vi "Temperature viewer.vi"(3 "ChipID+T array":u32[](array[numeric]) format="%.0x") -> ()   [LabVIEW 2015, in "VIPM2.lvlib"]
uses:
  VIPM2.lvlib
panel:
  out "S18 Chart":sgl(graph)
  out "S18 histogram":T1(graph) caption="Temperature histogram"
  out "S17 Chart":sgl(graph)
  out "S17 histogram":T1(graph) caption="Temperature histogram"
  out "S16 Chart":sgl(graph)
  out "S16 histogram":T1(graph) caption="Temperature histogram"
  out "S15 Chart":sgl(graph)
  out "S15 histogram":T1(graph) caption="Temperature histogram"
  out "S14 Chart":sgl(graph)
  out "S14 histogram":T1(graph) caption="Temperature histogram"
  out "S13 Chart":sgl(graph)
  out "S13 histogram":T1(graph) caption="Temperature histogram"
  out "S12 Chart":sgl(graph)
  out "S12 histogram":T1(graph) caption="Temperature histogram"
  out "S11 Chart":sgl(graph)
  out "S11 histogram":T1(graph) caption="Temperature histogram"
  out "S10 Chart":sgl(graph)
  out "S10 histogram":T1(graph) caption="Temperature histogram"
  out "S09 Chart":sgl(graph)
  out "S09 histogram":T1(graph) caption="Temperature histogram"
  out "S08 Chart":sgl(graph)
  out "S08 histogram":T1(graph) caption="Temperature histogram"
  out "S07 Chart":sgl(graph)
  out "S07 histogram":T1(graph) caption="Temperature histogram"
  out "S06 Chart":sgl(graph)
  out "S06 histogram":T1(graph) caption="Temperature histogram"
  out "S05 Chart":sgl(graph)
  out "S05 histogram":T1(graph) caption="Temperature histogram"
  out "S04 Chart":sgl(graph)
  out "S04 histogram":T1(graph) caption="Temperature histogram"
  out "S03 Chart":sgl(graph)
  out "S03 histogram":T1(graph) caption="Temperature histogram"
  out "S02 Chart":sgl(graph)
  out "S02 histogram":T1(graph) caption="Temperature histogram"
  out "S01 Chart":sgl(graph)
  out "S01 histogram":T1(graph) caption="Temperature histogram"
  # "Sector 01"
  # "Sector 02"
  # "Sector 03"
  # "Sector 04"
  # "Sector 05"
  # "Sector 06"
  # "Sector 07"
  # "Sector 08"
  # "Sector 09"
  # "Sector 10"
  # "Sector 11"
  # "Sector 12"
  # "Sector 13"
  # "Sector 14"
  # "Sector 15"
  # "Sector 16"
  # "Sector 17"
  # "Sector 18"
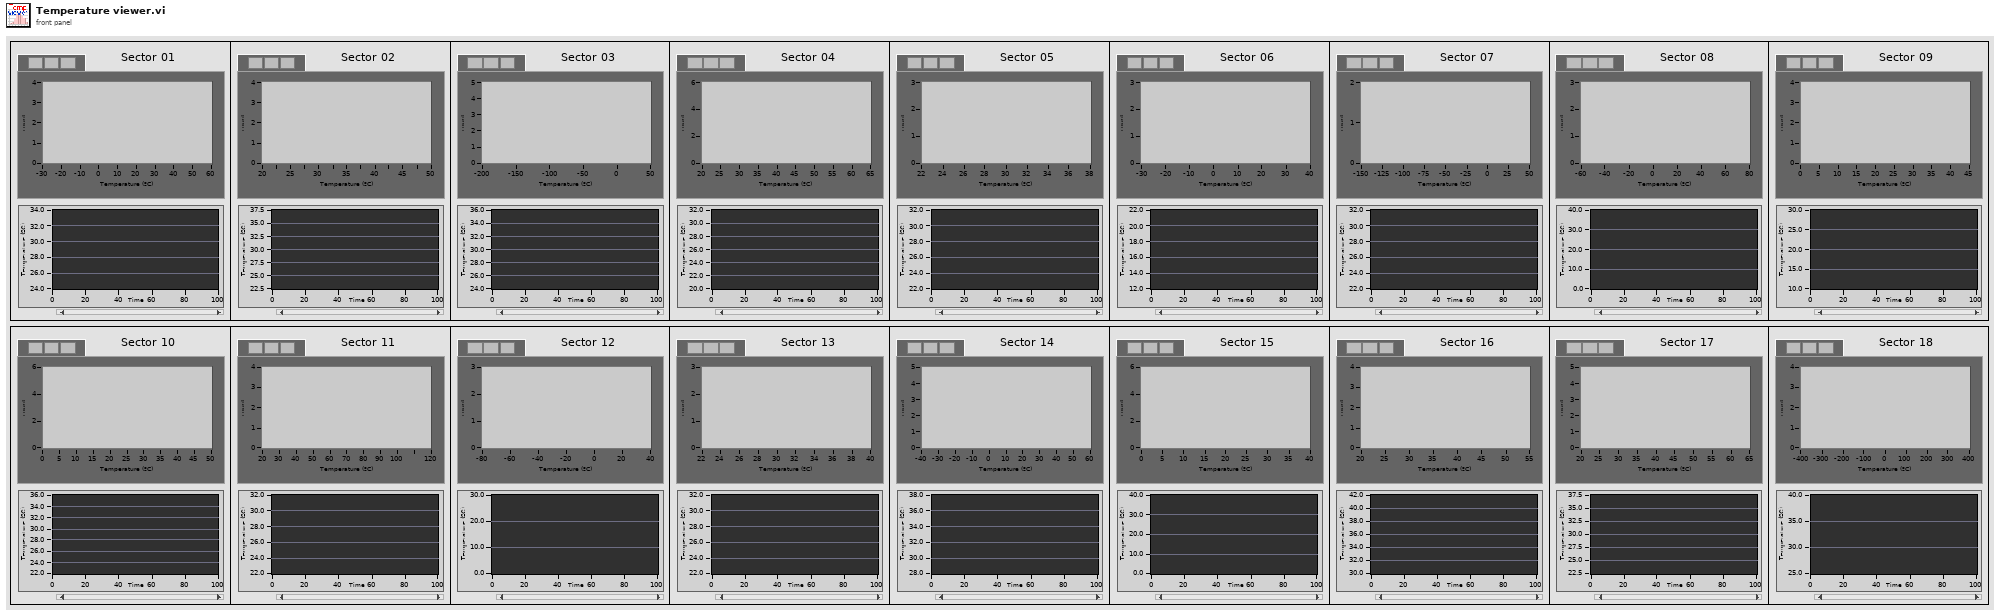
[diagram p1: front panel]
types:
  T1 = cluster{"X Values":dbl[], "Histogram: h(x)":i32[]}
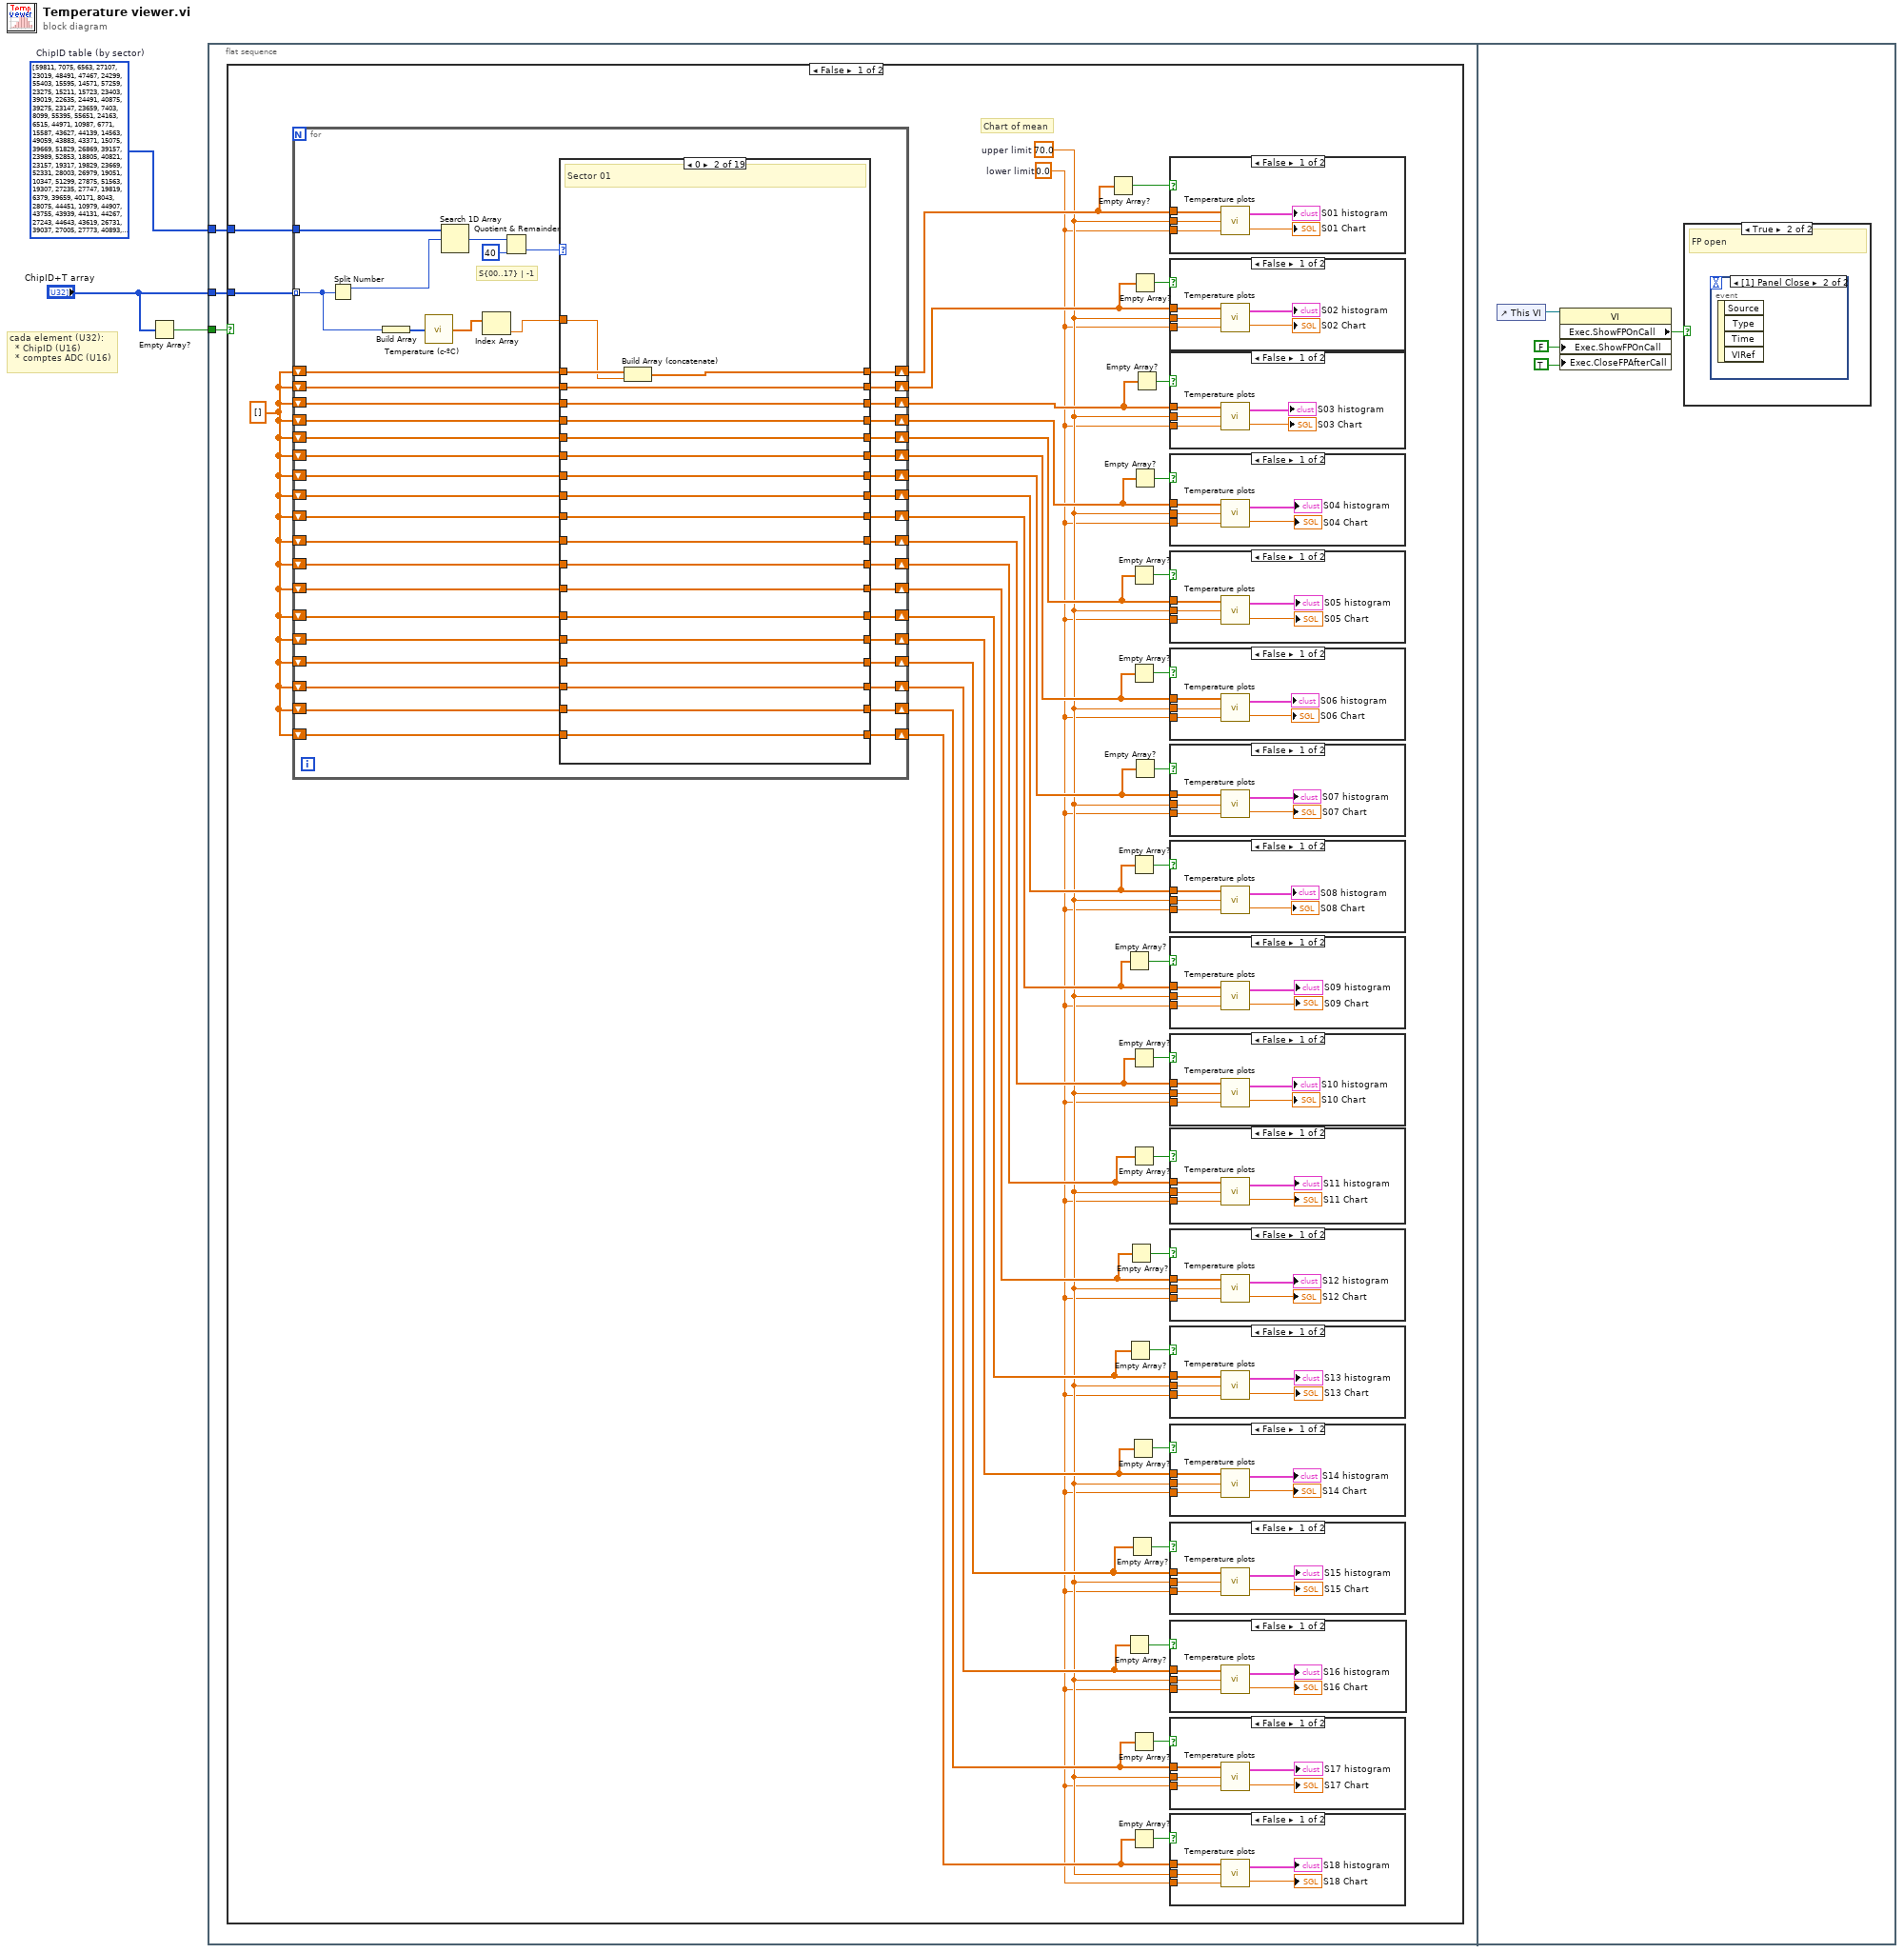
[diagram p0: block diagram]
diagram:
  w2 = u16[] [59811, 7075, 6563, 27107, 23019, 48491, 47467, 24299, 55403, 15595, 14571, 57259, 23275, 15211, 15723, 23403, 39019, 22635, 24491, 40875, 39275, 23147, 23659, 7403, 8099, 55395, 55651, 24163, 6515, 44971, 10987, 6771, 15587, 43627, 44139, 14563, 49059, 43883, 43371, 15075, 39669, 51829, 26869, 39157, 23989, 52853, 18805, 40821, 23157, 19317, 19829, 23669, 52331, 28003, 26979, 19051, 10347, 51299, 27875, 51563, 19307, 27235, 27747, 19819, 6379, 39659, 40171, 8043, 28075, 44451, 10979, 44907, 43755, 43939, 44131, 44267, 27243, 44643, 43619, 26731, 39037, 27005, 27773, 40893, 40189, 27517, 28029, 39165, 56165, 60645, 59621, 56677, 55525, 60261, 60517, 57189, 48357, 60773, 61349, 47333, 61309, 14461, 16317, 60797, 6525, 14965, 24189, 8125, 31845, 7781, 8101, 47845, 60669, 55805, 56061, 59773, 47973, 6245, 61157, 16229, 60541, 56765, 23037, 59517, 6589, 56445, 57277, 59901, 61181, 55549, 57213, 61373, 23485, 28285, 43133, 23997, 23677, 43965, 44477, 24509, 26877, 23293, 23805, 28541, 6765, 57261, 23789, 7085, 6509, 56941, 55917, 7789, 43629, 56045, 55661, 7533, 39421, 27581, 44925, 40317, 44269, 15469, 16301, 43245, 22627, 43261, 43645, 23971, 39549, 43389, 44669, 8035, 39293, 43773, 44285, 40573, 27885, 15603, 14579, 26861, 19309, 49075, 15731, 19821, 52845, 31859, 47859, 18797, 16125, 40867, 39843, 15101, 40675, 7421, 6397, 40291, 40163, 7037, 44157, 40803, 60269, 23021, 23405, 60781, 60141, 22765, 56429, 61293, 40805, 15741, 14717, 40037, 40165, 47869, 48381, 39141, 40677, 30973, 16253, 39653, 23141, 40035, 32381, 23461, 8037, 40547, 39523, 7013, 15613, 7907, 6883, 15997, 44397, 56173, 56685, 43373, 44909, 15277, 55789, 11501, 51835, 20071, 11003, 20091, 11195, 10491, 11131, 52603, 51451, 11643, 10619, 53115, 40827, 27239, 28263, 47207, 39291, 43111, 28071, 39803, 40059, 44391, 43879, 39547, 44661, 52469, 19061, 43637, 43957, 51445, 53109, 44469, 10997, 52597, 51573, 39797, 31341, 61037, 60013, 31853, 61051, 6267, 8123, 60027, 39867, 43623, 44647, 39035, 40379, 11495, 44135, 7931, 8059, 44455, 43943, 6395, 59835, 7099, 6587, 61371, 27131, 60155, 59899, 27387, 6375, 39655, 48359, 8039, 47847, 31335, 32359, 47335, 15975, 48743, 1120, 14951, 15719, 15079, 14567, 14695, 43387, 28282, 27259, 44667, 43899, 28027, 27003, 44411, 52333, 14949, 47347, 51309, 15973, 11879, 11367, 96, 31589, 60325, 60837, 31333, 14565, 15589, 15205, 14693, 43259, 28539, 27515, 44923, 3879, 57191, 56167, 57255, 55527, 56551, 15271, 14439, 31591, 23271, 23783, 31079, 60795, 7803, 6779, 59771, 61307, 7547, 6523, 60283, 26983, 61287, 59879, 28007, 26727, 6567, 8103, 26855, 59623, 7271, 39163, 59815, 40359, 23975, 39399, 39335, 40551, 22631, 24487, 39783, 39847, 23655, 23143, 39271, 60519, 40187, 39675, 60007, 27367, 24507, 23675, 60263, 27499, 44387, 43363, 26987, 26859, 28579, 44899, 28523, 57203, 39155, 40819, 56179, 56563, 39667, 40179, 55539, 15283, 39411, 40691, 57075, 56939, 47339, 48235, 56747, 55531, 31851, 48363, 56171, 44987, 43771, 44283, 43963, 43643, 28091, 26747, 44155, 15275, 31083, 32363, 55787, 59827, 48355, 47331, 27123, 61043, 31843, 47843, 60019, 60323, 7267, 6243, 60835, 59491, 6499, 7779, 27363, 39787, 59755, 61035, 40299, 23267, 56675, 57187, 23395, 22755, 55523, 56035, 24419, 55715, 57059, 40811, 24291, 23781, 56037, 56549, 22885, 39845, 48765, 47741, 416, 60147, 31075, 48995, 60659, 15725, 10365, 12221, 14701, 47213, 11197, 51453, 49069, 19815, 10343, 52455, 18791, 52071, 11111, 11623, 52839, 39269, 47997, 48509, 40549, 7525, 49021, 48253, 6501, 40373, 26741, 28597, 39349, 40885, 43893, 43381, 39861, 39285, 28021, 44917, 40053, 15597, 11133, 10877, 14957, 51437, 49011, 48243, 53101, 10605, 48755, 47731, 11885, 31603, 57267, 23795, 32115, 56755, 39795, 40307, 24307, 55667, 23475, 60339, 55923, 11637, 32109, 31085, 10613, 12149, 52093, 31597, 11125, 16237, 19325, 18813, 15213, 6387, 22643, 24499, 14451, 7923, 23155, 23667, 6899, 16227, 47459, 48739, 14691, 10477, 47987, 47219, 12141, 24435, 40369, 39347, 23411, 31091, 30963, 32627, 32371, 47981, 10621, 11901, 48493, 47341, 10493, 12157, 48237, 47853, 60845, 27373, 48365, 31349, 15285, 55797, 31861, 60661, 56949, 55925, 59637, 59765, 56053, 55669, 48373, 60341, 56693, 23797, 60853, 59509, 23029, 24309, 61365, 60277, 23925, 23413, 60789, 31093, 6261, 60533, 32373, 31605, 6517, 6773, 32117, 30965, 15477, 14453, 32629, 7925, 44277, 43253, 6901, 40363, 39403, 40683, 39339, 6581, 7029, 8053, 59893, 60349, 47349, 49013, 6269, 27133, 16117, 48757, 27389, 24445, 47989, 47221, 23933, 26867, 31587, 32099, 60787, 7091, 30947, 32611, 59891, 7539, 47203, 11499, 6259, 28013, 16243, 15219, 26989, 28525, 14963, 11117, 28589, 28077, 12205, 52461, 27245, 55909, 61029, 60005, 57253, 23397, 14437, 16293, 23909, 55653, 60133, 59749, 56933, 10475, 51811, 19043, 11883, 10859, 52067, 51555, 11491, 51427, 60003, 60515, 52451, 23915, 14699, 15979, 22891, 60331, 16107, 15459, 61291, 39531, 60139, 60651, 40043, 10595, 60643, 59619, 11875, 11363, 60259, 61027, 12195]  # ChipID table (by sector)
  # "cada element (U32):\n  * ChipID (U16)\n  * comptes ADC (U16)"
  n1 = Empty Array?(array="ChipID+T array") -> (empty?=w1:bool)
  n2 = flat-sequence {
    tunnel: "ChipID+T array" -> [w6]
    tunnel: w2 -> [w5]
    tunnel: w1 -> [w4]
    frame #0 {
      n3 = case shown="False" w4 {
        tunnel: w6 -> [w47 _]
        tunnel: w5 -> [w46 _]
        frame False {
          w8 = sgl 70.0  # upper limit
          w7 = sgl 0.0  # lower limit
          w42 = sgl[] []
          # "Chart of mean"
          n4 = for {
            tunnel: w47 -> [w141] mode=indexing
            tunnel: w46 -> [w181]
            shift-right: [w179] -> w45
            shift-left: w42 -> [w180]
            shift-right: [w174] -> w41
            shift-left: w42 -> [w178]
            shift-right: [w173] -> w39
            shift-left: w42 -> [w177]
            shift-right: [w172] -> w37
            shift-left: w42 -> [w176]
            shift-right: [w171] -> w35
            shift-left: w42 -> [w175]
            shift-right: [w154] -> w33
            shift-left: w42 -> [w167]
            shift-right: [w153] -> w31
            shift-left: w42 -> [w166]
            shift-right: [w152] -> w29
            shift-left: w42 -> [w165]
            shift-right: [w151] -> w27
            shift-left: w42 -> [w164]
            shift-right: [w150] -> w25
            shift-left: w42 -> [w163]
            shift-right: [w149] -> w23
            shift-left: w42 -> [w162]
            shift-right: [w148] -> w21
            shift-left: w42 -> [w161]
            shift-right: [w147] -> w19
            shift-left: w42 -> [w160]
            shift-right: [w146] -> w17
            shift-left: w42 -> [w159]
            shift-right: [w145] -> w15
            shift-left: w42 -> [w158]
            shift-right: [w144] -> w13
            shift-left: w42 -> [w157]
            shift-right: [w143] -> w11
            shift-left: w42 -> [w156]
            shift-right: [w142] -> w9
            shift-left: w42 -> [w155]
            # "S{00..17} | -1"
            n5 = Split Number(x=w141) -> (hi(x)=w182:u16)  [unwired: 1 out]
            n6 = Build Array(w141) -> (w140:u32[])
            n7 = call "Temperature (c-ºC).vi"("ChipID + Tcounts"=w140) -> ("Temperatures in ºC"=w139:sgl[])  [unwired: 3 in]
            n8 = Search 1D Array(1D array=w181, element=w182) -> (index of element=w170:i32)  [unwired: 1 in]
            n9 = Index Array(array=w139) -> (element=w138:sgl)  [unwired: 1 in]
            n10 = Quotient & Remainder(x=w170, y=40) -> (floor(x/y)=w168:i32)  [unwired: 1 out]
            n11 = case shown="0" w168 {
              tunnel: w138 -> [_ w219 w238 w257 w276 w295 w314 w333 w352 w371 w390 w409 w428 w447 w466 w485 w504 w523 w542]
              tunnel: w180 -> [w200 w220 w240 w260 w280 w300 w320 w340 w360 w380 w400 w420 w440 w460 w480 w500 w520 w540 w560]
              tunnel: [w200 w218 w240 w260 w280 w300 w320 w340 w360 w380 w400 w420 w440 w460 w480 w500 w520 w540 w560] -> w179
              tunnel: w178 -> [w199 w217 w239 w259 w279 w299 w319 w339 w359 w379 w399 w419 w439 w459 w479 w499 w519 w539 w559]
              tunnel: w177 -> [w198 w216 w236 w258 w278 w298 w318 w338 w358 w378 w398 w418 w438 w458 w478 w498 w518 w538 w558]
              tunnel: w176 -> [w197 w215 w235 w255 w277 w297 w317 w337 w357 w377 w397 w417 w437 w457 w477 w497 w517 w537 w557]
              tunnel: w175 -> [w196 w214 w234 w254 w274 w296 w316 w336 w356 w376 w396 w416 w436 w456 w476 w496 w516 w536 w556]
              tunnel: [w199 w217 w237 w259 w279 w299 w319 w339 w359 w379 w399 w419 w439 w459 w479 w499 w519 w539 w559] -> w174
              tunnel: [w198 w216 w236 w256 w278 w298 w318 w338 w358 w378 w398 w418 w438 w458 w478 w498 w518 w538 w558] -> w173
              tunnel: [w197 w215 w235 w255 w275 w297 w317 w337 w357 w377 w397 w417 w437 w457 w477 w497 w517 w537 w557] -> w172
              tunnel: [w196 w214 w234 w254 w274 w294 w316 w336 w356 w376 w396 w416 w436 w456 w476 w496 w516 w536 w556] -> w171
              tunnel: w167 -> [w195 w213 w233 w253 w273 w293 w315 w335 w355 w375 w395 w415 w435 w455 w475 w495 w515 w535 w555]
              tunnel: w166 -> [w194 w212 w232 w252 w272 w292 w312 w334 w354 w374 w394 w414 w434 w454 w474 w494 w514 w534 w554]
              tunnel: w165 -> [w193 w211 w231 w251 w271 w291 w311 w331 w353 w373 w393 w413 w433 w453 w473 w493 w513 w533 w553]
              tunnel: w164 -> [w192 w210 w230 w250 w270 w290 w310 w330 w350 w372 w392 w412 w432 w452 w472 w492 w512 w532 w552]
              tunnel: w163 -> [w191 w209 w229 w249 w269 w289 w309 w329 w349 w369 w391 w411 w431 w451 w471 w491 w511 w531 w551]
              tunnel: w162 -> [w190 w208 w228 w248 w268 w288 w308 w328 w348 w368 w388 w410 w430 w450 w470 w490 w510 w530 w550]
              tunnel: w161 -> [w189 w207 w227 w247 w267 w287 w307 w327 w347 w367 w387 w407 w429 w449 w469 w489 w509 w529 w549]
              tunnel: w160 -> [w188 w206 w226 w246 w266 w286 w306 w326 w346 w366 w386 w406 w426 w448 w468 w488 w508 w528 w548]
              tunnel: w159 -> [w187 w205 w225 w245 w265 w285 w305 w325 w345 w365 w385 w405 w425 w445 w467 w487 w507 w527 w547]
              tunnel: w158 -> [w186 w204 w224 w244 w264 w284 w304 w324 w344 w364 w384 w404 w424 w444 w464 w486 w506 w526 w546]
              tunnel: w157 -> [w185 w203 w223 w243 w263 w283 w303 w323 w343 w363 w383 w403 w423 w443 w463 w483 w505 w525 w545]
              tunnel: w156 -> [w184 w202 w222 w242 w262 w282 w302 w322 w342 w362 w382 w402 w422 w442 w462 w482 w502 w524 w544]
              tunnel: w155 -> [w183 w201 w221 w241 w261 w281 w301 w321 w341 w361 w381 w401 w421 w441 w461 w481 w501 w521 w543]
              tunnel: [w195 w213 w233 w253 w273 w293 w313 w335 w355 w375 w395 w415 w435 w455 w475 w495 w515 w535 w555] -> w154
              tunnel: [w194 w212 w232 w252 w272 w292 w312 w332 w354 w374 w394 w414 w434 w454 w474 w494 w514 w534 w554] -> w153
              tunnel: [w193 w211 w231 w251 w271 w291 w311 w331 w351 w373 w393 w413 w433 w453 w473 w493 w513 w533 w553] -> w152
              tunnel: [w192 w210 w230 w250 w270 w290 w310 w330 w350 w370 w392 w412 w432 w452 w472 w492 w512 w532 w552] -> w151
              tunnel: [w191 w209 w229 w249 w269 w289 w309 w329 w349 w369 w389 w411 w431 w451 w471 w491 w511 w531 w551] -> w150
              tunnel: [w190 w208 w228 w248 w268 w288 w308 w328 w348 w368 w388 w408 w430 w450 w470 w490 w510 w530 w550] -> w149
              tunnel: [w189 w207 w227 w247 w267 w287 w307 w327 w347 w367 w387 w407 w427 w449 w469 w489 w509 w529 w549] -> w148
              tunnel: [w188 w206 w226 w246 w266 w286 w306 w326 w346 w366 w386 w406 w426 w446 w468 w488 w508 w528 w548] -> w147
              tunnel: [w187 w205 w225 w245 w265 w285 w305 w325 w345 w365 w385 w405 w425 w445 w465 w487 w507 w527 w547] -> w146
              tunnel: [w186 w204 w224 w244 w264 w284 w304 w324 w344 w364 w384 w404 w424 w444 w464 w484 w506 w526 w546] -> w145
              tunnel: [w185 w203 w223 w243 w263 w283 w303 w323 w343 w363 w383 w403 w423 w443 w463 w483 w503 w525 w545] -> w144
              tunnel: [w184 w202 w222 w242 w262 w282 w302 w322 w342 w362 w382 w402 w422 w442 w462 w482 w502 w522 w544] -> w143
              tunnel: [w183 w201 w221 w241 w261 w281 w301 w321 w341 w361 w381 w401 w421 w441 w461 w481 w501 w521 w541] -> w142
              frame -1, Default {
                # "ChipID not found"
              }
              frame 0 {
                # "Sector 01"
                n12 = Build Array (concatenate) "Build Array"(w220, w219) -> (w218:sgl[])
              }
              frame 1 {
                # "Sector 02"
                n13 = Build Array (concatenate)(w239, w238) -> (w237:sgl[])
              }
              frame 2 {
                # "Sector 03"
                n14 = Build Array (concatenate)(w258, w257) -> (w256:sgl[])
              }
              frame 3 {
                # "Sector 04"
                n15 = Build Array (concatenate)(w277, w276) -> (w275:sgl[])
              }
              frame 4 {
                # "Sector 05"
                n16 = Build Array (concatenate)(w296, w295) -> (w294:sgl[])
              }
              frame 5 {
                # "Sector 06"
                n17 = Build Array (concatenate)(w315, w314) -> (w313:sgl[])
              }
              frame 6 {
                # "Sector 07"
                n18 = Build Array (concatenate)(w334, w333) -> (w332:sgl[])
              }
              frame 7 {
                # "Sector 08"
                n19 = Build Array (concatenate)(w353, w352) -> (w351:sgl[])
              }
              frame 8 {
                # "Sector 09"
                n20 = Build Array (concatenate)(w372, w371) -> (w370:sgl[])
              }
              frame 9 {
                # "Sector 10"
                n21 = Build Array (concatenate)(w391, w390) -> (w389:sgl[])
              }
              frame 10 {
                # "Sector 11"
                n22 = Build Array (concatenate)(w410, w409) -> (w408:sgl[])
              }
              frame 11 {
                # "Sector 12"
                n23 = Build Array (concatenate)(w429, w428) -> (w427:sgl[])
              }
              frame 12 {
                # "Sector 13"
                n24 = Build Array (concatenate)(w448, w447) -> (w446:sgl[])
              }
              frame 13 {
                # "Sector 14"
                n25 = Build Array (concatenate)(w467, w466) -> (w465:sgl[])
              }
              frame 14 {
                # "Sector 15"
                n26 = Build Array (concatenate)(w486, w485) -> (w484:sgl[])
              }
              frame 15 {
                # "Sector 16"
                n27 = Build Array (concatenate)(w505, w504) -> (w503:sgl[])
              }
              frame 16 {
                # "Sector 17"
                n28 = Build Array (concatenate)(w524, w523) -> (w522:sgl[])
              }
              frame 17 {
                # "Sector 18"
                n29 = Build Array (concatenate)(w543, w542) -> (w541:sgl[])
              }
            }
          }
          n30 = Empty Array?(array=w45) -> (empty?=w44:bool)
          n31 = Empty Array?(array=w27) -> (empty?=w28:bool)
          n32 = Empty Array?(array=w13) -> (empty?=w14:bool)
          n33 = Empty Array?(array=w19) -> (empty?=w20:bool)
          n34 = Empty Array?(array=w21) -> (empty?=w22:bool)
          n35 = Empty Array?(array=w15) -> (empty?=w16:bool)
          n36 = Empty Array?(array=w17) -> (empty?=w18:bool)
          n37 = Empty Array?(array=w35) -> (empty?=w36:bool)
          n38 = Empty Array?(array=w33) -> (empty?=w34:bool)
          n39 = Empty Array?(array=w29) -> (empty?=w30:bool)
          n40 = Empty Array?(array=w25) -> (empty?=w26:bool)
          n41 = Empty Array?(array=w23) -> (empty?=w24:bool)
          n42 = Empty Array?(array=w11) -> (empty?=w12:bool)
          n43 = Empty Array?(array=w9) -> (empty?=w10:bool)
          n44 = Empty Array?(array=w41) -> (empty?=w43:bool)
          n45 = Empty Array?(array=w37) -> (empty?=w38:bool)
          n46 = Empty Array?(array=w31) -> (empty?=w32:bool)
          n47 = Empty Array?(array=w39) -> (empty?=w40:bool)
          n48 = case shown="False" w44 {
            tunnel: w45 -> [w137 _]
            tunnel: w8 -> [w136 _]
            tunnel: w7 -> [w135 _]
            frame False {
              n49 = call "Temperature plots.vi"("lower limit"=w135, "upper limit"=w136, "Temperatures"=w137) -> ("Sxx Chart"=→"S01 Chart":sgl, "Sxx histogram"=→"S01 histogram":T1)  [unwired: 1 in]
            }
            frame True {
            }
          }
          n50 = case shown="False" w43 {
            tunnel: w41 -> [w132 _]
            tunnel: w8 -> [w131 _]
            tunnel: w7 -> [w130 _]
            frame False {
              n51 = call "Temperature plots.vi"("lower limit"=w130, "upper limit"=w131, "Temperatures"=w132) -> ("Sxx Chart"=→"S02 Chart":sgl, "Sxx histogram"=→"S02 histogram":T1)  [unwired: 1 in]
            }
            frame True {
            }
          }
          n52 = case shown="False" w40 {
            tunnel: w39 -> [w127 _]
            tunnel: w8 -> [w126 _]
            tunnel: w7 -> [w125 _]
            frame False {
              n53 = call "Temperature plots.vi"("lower limit"=w125, "upper limit"=w126, "Temperatures"=w127) -> ("Sxx Chart"=→"S03 Chart":sgl, "Sxx histogram"=→"S03 histogram":T1)  [unwired: 1 in]
            }
            frame True {
            }
          }
          n54 = case shown="False" w38 {
            tunnel: w37 -> [w122 _]
            tunnel: w8 -> [w121 _]
            tunnel: w7 -> [w120 _]
            frame False {
              n55 = call "Temperature plots.vi"("lower limit"=w120, "upper limit"=w121, "Temperatures"=w122) -> ("Sxx Chart"=→"S04 Chart":sgl, "Sxx histogram"=→"S04 histogram":T1)  [unwired: 1 in]
            }
            frame True {
            }
          }
          n56 = case shown="False" w36 {
            tunnel: w35 -> [w117 _]
            tunnel: w8 -> [w116 _]
            tunnel: w7 -> [w115 _]
            frame False {
              n57 = call "Temperature plots.vi"("lower limit"=w115, "upper limit"=w116, "Temperatures"=w117) -> ("Sxx Chart"=→"S05 Chart":sgl, "Sxx histogram"=→"S05 histogram":T1)  [unwired: 1 in]
            }
            frame True {
            }
          }
          n58 = case shown="False" w34 {
            tunnel: w33 -> [w112 _]
            tunnel: w8 -> [w111 _]
            tunnel: w7 -> [w110 _]
            frame False {
              n59 = call "Temperature plots.vi"("lower limit"=w110, "upper limit"=w111, "Temperatures"=w112) -> ("Sxx Chart"=→"S06 Chart":sgl, "Sxx histogram"=→"S06 histogram":T1)  [unwired: 1 in]
            }
            frame True {
            }
          }
          n60 = case shown="False" w32 {
            tunnel: w31 -> [w107 _]
            tunnel: w8 -> [w106 _]
            tunnel: w7 -> [w105 _]
            frame False {
              n61 = call "Temperature plots.vi"("lower limit"=w105, "upper limit"=w106, "Temperatures"=w107) -> ("Sxx Chart"=→"S07 Chart":sgl, "Sxx histogram"=→"S07 histogram":T1)  [unwired: 1 in]
            }
            frame True {
            }
          }
          n62 = case shown="False" w30 {
            tunnel: w29 -> [w102 _]
            tunnel: w8 -> [w101 _]
            tunnel: w7 -> [w100 _]
            frame False {
              n63 = call "Temperature plots.vi"("lower limit"=w100, "upper limit"=w101, "Temperatures"=w102) -> ("Sxx Chart"=→"S08 Chart":sgl, "Sxx histogram"=→"S08 histogram":T1)  [unwired: 1 in]
            }
            frame True {
            }
          }
          n64 = case shown="False" w28 {
            tunnel: w27 -> [w97 _]
            tunnel: w8 -> [w96 _]
            tunnel: w7 -> [w95 _]
            frame False {
              n65 = call "Temperature plots.vi"("lower limit"=w95, "upper limit"=w96, "Temperatures"=w97) -> ("Sxx Chart"=→"S09 Chart":sgl, "Sxx histogram"=→"S09 histogram":T1)  [unwired: 1 in]
            }
            frame True {
            }
          }
          n66 = case shown="False" w26 {
            tunnel: w25 -> [w92 _]
            tunnel: w8 -> [w91 _]
            tunnel: w7 -> [w90 _]
            frame False {
              n67 = call "Temperature plots.vi"("lower limit"=w90, "upper limit"=w91, "Temperatures"=w92) -> ("Sxx Chart"=→"S10 Chart":sgl, "Sxx histogram"=→"S10 histogram":T1)  [unwired: 1 in]
            }
            frame True {
            }
          }
          n68 = case shown="False" w24 {
            tunnel: w23 -> [w87 _]
            tunnel: w8 -> [w86 _]
            tunnel: w7 -> [w85 _]
            frame False {
              n69 = call "Temperature plots.vi"("lower limit"=w85, "upper limit"=w86, "Temperatures"=w87) -> ("Sxx Chart"=→"S11 Chart":sgl, "Sxx histogram"=→"S11 histogram":T1)  [unwired: 1 in]
            }
            frame True {
            }
          }
          n70 = case shown="False" w22 {
            tunnel: w21 -> [w82 _]
            tunnel: w8 -> [w81 _]
            tunnel: w7 -> [w80 _]
            frame False {
              n71 = call "Temperature plots.vi"("lower limit"=w80, "upper limit"=w81, "Temperatures"=w82) -> ("Sxx Chart"=→"S12 Chart":sgl, "Sxx histogram"=→"S12 histogram":T1)  [unwired: 1 in]
            }
            frame True {
            }
          }
          n72 = case shown="False" w20 {
            tunnel: w19 -> [w77 _]
            tunnel: w8 -> [w76 _]
            tunnel: w7 -> [w75 _]
            frame False {
              n73 = call "Temperature plots.vi"("lower limit"=w75, "upper limit"=w76, "Temperatures"=w77) -> ("Sxx Chart"=→"S13 Chart":sgl, "Sxx histogram"=→"S13 histogram":T1)  [unwired: 1 in]
            }
            frame True {
            }
          }
          n74 = case shown="False" w18 {
            tunnel: w17 -> [w72 _]
            tunnel: w8 -> [w71 _]
            tunnel: w7 -> [w70 _]
            frame False {
              n75 = call "Temperature plots.vi"("lower limit"=w70, "upper limit"=w71, "Temperatures"=w72) -> ("Sxx Chart"=→"S14 Chart":sgl, "Sxx histogram"=→"S14 histogram":T1)  [unwired: 1 in]
            }
            frame True {
            }
          }
          n76 = case shown="False" w16 {
            tunnel: w15 -> [w67 _]
            tunnel: w8 -> [w66 _]
            tunnel: w7 -> [w65 _]
            frame False {
              n77 = call "Temperature plots.vi"("lower limit"=w65, "upper limit"=w66, "Temperatures"=w67) -> ("Sxx Chart"=→"S15 Chart":sgl, "Sxx histogram"=→"S15 histogram":T1)  [unwired: 1 in]
            }
            frame True {
            }
          }
          n78 = case shown="False" w14 {
            tunnel: w13 -> [w62 _]
            tunnel: w8 -> [w61 _]
            tunnel: w7 -> [w60 _]
            frame False {
              n79 = call "Temperature plots.vi"("lower limit"=w60, "upper limit"=w61, "Temperatures"=w62) -> ("Sxx Chart"=→"S16 Chart":sgl, "Sxx histogram"=→"S16 histogram":T1)  [unwired: 1 in]
            }
            frame True {
            }
          }
          n80 = case shown="False" w12 {
            tunnel: w11 -> [w57 _]
            tunnel: w8 -> [w56 _]
            tunnel: w7 -> [w55 _]
            frame False {
              n81 = call "Temperature plots.vi"("lower limit"=w55, "upper limit"=w56, "Temperatures"=w57) -> ("Sxx Chart"=→"S17 Chart":sgl, "Sxx histogram"=→"S17 histogram":T1)  [unwired: 1 in]
            }
            frame True {
            }
          }
          n82 = case shown="False" w10 {
            tunnel: w9 -> [w52 _]
            tunnel: w8 -> [w51 _]
            tunnel: w7 -> [w50 _]
            frame False {
              n83 = call "Temperature plots.vi"("lower limit"=w50, "upper limit"=w51, "Temperatures"=w52) -> ("Sxx Chart"=→"S18 Chart":sgl, "Sxx histogram"=→"S18 histogram":T1)  [unwired: 1 in]
            }
            frame True {
            }
          }
        }
        frame True {
        }
      }
    }
    frame #1 {
      n84 = control-ref of="This VI"() -> (w562:refnum<vi>)
      n85 = property class="VI"(reference=w562, "Exec.ShowFPOnCall"=FALSE, "Exec.CloseFPAfterCall"=TRUE ("Execution:Close After Call")) -> ("Exec.ShowFPOnCall"=w561:bool)  [unwired: 1 in, 2 out]
      n86 = case shown="True" w561 {
        frame False {
          # "FP no open"
        }
        frame True {
          # "FP open"
          n87 = event shown="[1] Panel Close" {
            selector: _ -> [_ _]
            dyn-events: _ -> [_ _]
            timeout: _ -> [_ _]
            event Timeout {
              n88 = event-data() -> ()  [unwired: 1 in, 3 out]
            }
            event Panel Close {
              n89 = event-data() -> ()  [unwired: 1 in, 4 out]
            }
          }
        }
      }
    }
  }
